vi "N Field Set Text In.vi"(1 "command text in":string[](array[string])=["N/A", "Magent PS", "N/A", "Set Field", "Set Field to 2.0000E+0 @ 0.0000T /min, no wait , extra 0 sec wait", "N/A", "N/A", "", "1", "0", "N/A", "2.000000", "0.000000", "N/A", "N/A", "N/A", "N/A", "N/A", "N/A", "N/A", "N/A", "N/A", "N/A", "N/A", "N/A", "N/A", "N/A", "N/A", "N/A", "N/A", "N/A", "N/A", "N/A", "N/A"]) -> (0 "SetFieldCluster":T1={"rate"=0.0005, "set point"=0.0, "extra wait"=5, "wait option"=1} {"wait option" items=["Do not wait, just move on", "Wait until it reaches the set point."]; "extra wait" min=0; "set point" format="%.5f"; "rate" format="%.5f"})   [LabVIEW 2020]
uses:
  Field Set.ctl
panel:
  # "Set Field Command"
  # "T"
  # "at"
  # "T/min"
  # "1. Sweep field to"
  # "2. AND wait extra"
  # "seconds"
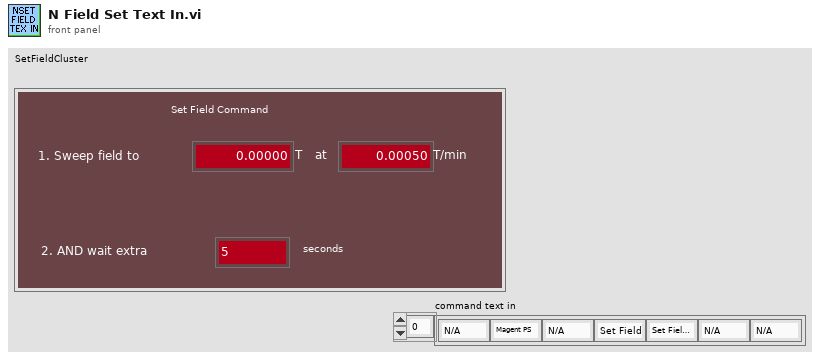
[diagram p1: front panel]
types:
  T1 = typedef "Field Set.ctl" = cluster{"rate":dbl, "set point":dbl, "extra wait":i32, "wait option":u16}
  T2 = cluster{"command text in[0]":string, "command text in[1]":string, "command text in[2]":string, "command text in[3]":string, "command text in[4]":string, "command text in[5]":string, "command text in[6]":string, "command text in[7]":string, "command text in[8]":string, "command text in[9]":string, "command text in[10]":string, "command text in[11]":string, "command text in[12]":string, "command text in[13]":string, "command text in[14]":string, "command text in[15]":string, "command text in[16]":string, "command text in[17]":string, "command text in[18]":string, "command text in[19]":string}
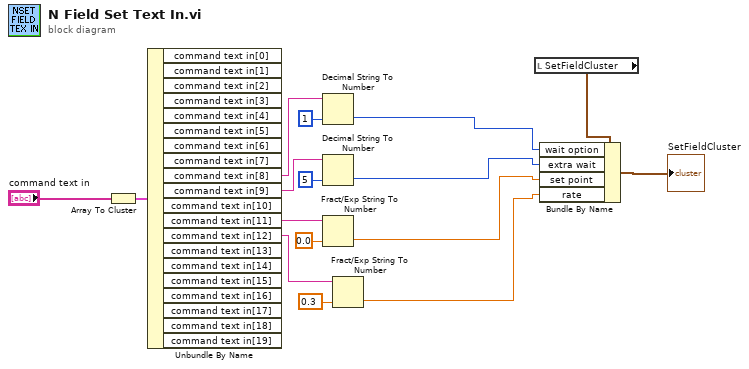
[diagram p0: block diagram]
diagram:
  n1 = Array To Cluster(array="command text in") -> (cluster=w15:T2)
  n2 = Unbundle By Name(w15) -> ("command text in[8]"=w14:string, "command text in[9]"=w13:string, "command text in[11]"=w12:string, "command text in[12]"=w11:string)  [unwired: 16 out]
  n3 = Decimal String To Number(string=w14, default (0L)=1 ("default (0 I32)")) -> (number=w4:i32)  [unwired: 1 in, 1 out]
  n4 = Decimal String To Number(string=w13, default (0L)=5 ("default (0 I32)")) -> (number=w3:i32)  [unwired: 1 in, 1 out]
  n5 = Fract/Exp String To Number(string=w12, default (0 dbl)=0.0 ("default (0 DBL)")) -> (number=w2:dbl)  [unwired: 2 in, 1 out]
  n6 = Fract/Exp String To Number(string=w11, default (0 dbl)=0.3 ("default (0 DBL)")) -> (number=w1:dbl)  [unwired: 2 in, 1 out]
  n7 = local read "SetFieldCluster"() -> (w6:T1)
  n8 = Bundle By Name(cluster=w6, "wait option"=w4, "extra wait"=w3, "set point"=w2, "rate"=w1) -> (→"SetFieldCluster":T1)
